vi "Ramp3.vi"(6 "# of Samples":dbl=201.0 format="%#_13g") -> (2 "Output":dbl[](array[numeric]))   [LabVIEW 2018]
panel:
  out "x+y":dbl
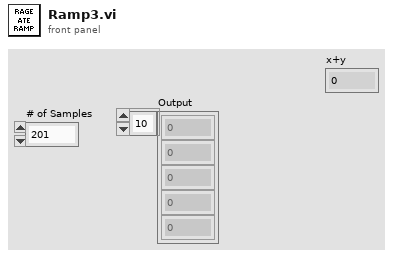
[diagram p1: front panel]
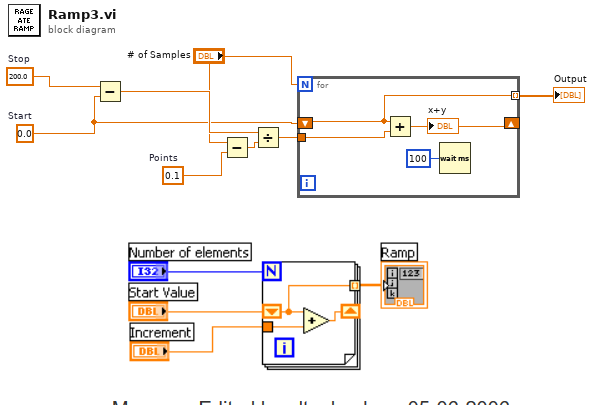
[diagram p0: block diagram]
diagram:
  w4 = 0.0  # Start
  w7 = 200.0  # Stop
  w1 = 0.1  # Points
  n1 = Subtract(x=w7, y=w4) -> (x-y=w6:dbl)
  n2 = Subtract(x="# of Samples", y=w1) -> (x-y=w3:dbl)
  n3 = Divide(x=w6, y=w3) -> (x/y=w5:dbl)
  n4 = for {
    N: "# of Samples" -> [_]
    shift-right: [w11] -> _
    shift-left: w4 -> [w12]
    tunnel: [w12] -> w8 mode=indexing
    tunnel: w5 -> [w10]
    n5 = Add(x=w12, y=w10) -> (x+y=w11:dbl)
    "x+y" <- w11
    n6 = Wait (ms)(milliseconds to wait=u32 100) -> ()  [unwired: 1 out]
  }
  "Output" <- w8
